vi "mod_sub_phase noise fit.vi"(0 "raw phase noise in":dbl[](array[numeric]) format="%.2f", 3 "f0":dbl=100.0 format="%.2f", 4 "error in (no error)":errorcluster, 5 "df":dbl=99.99921875610347 format="%.2f", 6 "polynomial order":i32=5, 7 "Section at what multiples?":dbl=10.0 format="%.2f", 9 "multiple buffer?":dbl=2.0 format="%.2f") -> (14 "phase noise fit":dbl[](array[numeric]) format="%.2f", 17 "phase noise plots":T1(array[cluster]) {"phase noise" format="%.2f"; "Ramp Pattern" format="%.2f"}, 19 "error out":errorcluster)   [LabVIEW 2020, in "niAMT.lvlib"]
uses:
  <vilib>/addons/Modulation/niAMT.lvlib
  <vilib>/Analysis/1siggen.llb/Ramp Pattern by Samples.vi
  <vilib>/measure/NI_MABase.lvlib
  <vilib>/Analysis/NI_AALBase.lvlib
  <vilib>/Analysis/NI_AALPro.lvlib
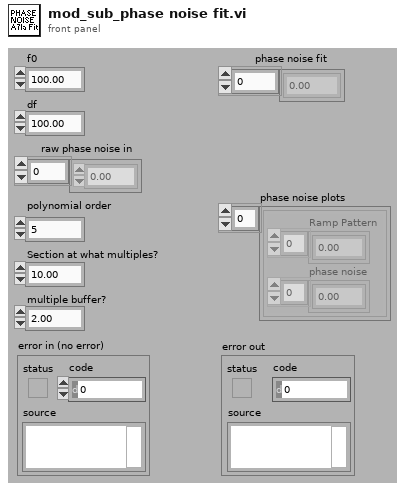
[diagram p1: front panel]
types:
  T1 = cluster{"Ramp Pattern":dbl[], "phase noise":dbl[]}[]
  T2 = enum32{"SVD", "Givens", "Givens2", "Householder", "LU Decomposition", "Cholesky"}
  T3 = cluster{"Ramp Pattern":dbl[], "raw phase noise in":dbl[]}
  T4 = cluster{"Ramp Pattern":dbl[], "raw phase noise in":dbl[]}[]
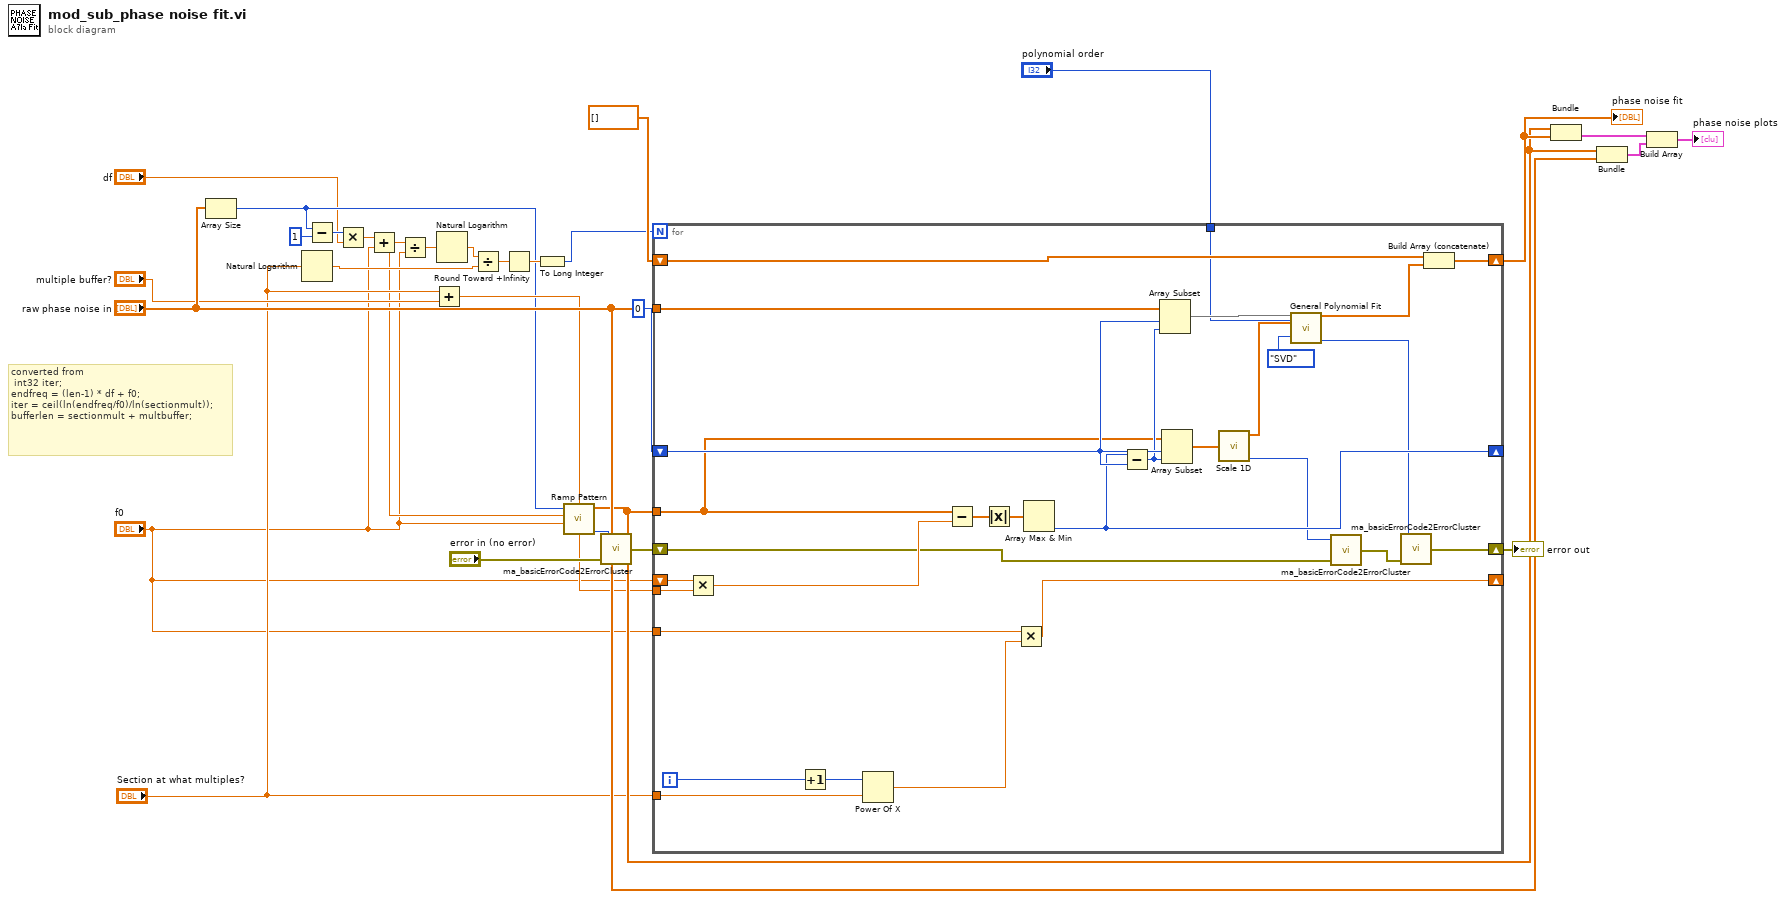
[diagram p0: block diagram]
diagram:
  # "converted from\n int32 iter;\nendfreq = (len-1) * df + f0;\niter = ceil(ln(endfreq/f0)/ln(sectionmult));\nbufferlen = sectionmult + multbuffer;"
  n1 = Array Size(array="raw phase noise in") -> (size(s)=w2:i32)
  n2 = Natural Logarithm(1:"Section at what multiples?") -> (0:w11:dbl)
  n3 = Subtract(x=w2, y=1) -> (x-y=w15:i32)
  n4 = Multiply(x=w15, y="df") -> (x*y=w14:dbl)
  n5 = Add(x=w14, y="f0") -> (x+y=w4:dbl)
  n6 = Divide(x=w4, y="f0") -> (x/y=w13:dbl)
  n7 = Add(x="Section at what multiples?", y="multiple buffer?") -> (x+y=w7:dbl)
  n8 = Natural Logarithm(1:w13) -> (0:w12:dbl)
  n9 = Divide(x=w12, y=w11) -> (x/y=w10:dbl)
  n10 = Round Toward +Infinity(x=w10) -> (ceil(x): smallest int >= x=w9:dbl)
  n11 = To Long Integer(number=w9) -> (32bit integer=w8:i32)
  n12 = call-poly <vilib>:"Ramp Pattern.vi"("start"="f0", "end"=w4, "samples"=w2) -> ("error"=w20:i32, "Ramp Pattern"=w21:dbl[])  [unwired: 7 in]
  n13 = call <vilib>:"ma_basicErrorCode2ErrorCluster.vi"("error in (no error)"="error in (no error)", "Error Code"=w20) -> ("error out"=w19:errorcluster)  [unwired: 1 in]
  n14 = for {
    N: w8 -> [_]
    shift-right: [w38] -> _
    shift-left: 0 -> [w54]
    tunnel: "raw phase noise in" -> [w55]
    tunnel: w21 -> [w45]
    tunnel: "Section at what multiples?" -> [w42]
    tunnel: "f0" -> [w58]
    tunnel: w7 -> [w56]
    shift-right: [w57] -> _
    shift-left: "f0" -> [w40]
    shift-right: [w49] -> w25
    shift-left: dbl[] [] -> [w48]
    tunnel: "polynomial order" -> [w36]
    shift-right: [w30] -> w18
    shift-left: w19 -> [w31]
    i -> [w44]
    n15 = Multiply(x=w40, y=w56) -> (x*y=w39:dbl)
    n16 = Increment(x=w44) -> (x+1=w43:i32)
    n17 = Power Of X(1:w42, 2:w43) -> (0:w41:dbl)
    n18 = Subtract(x=w45, y=w39) -> (x-y=w47:dbl[])
    n19 = Absolute Value(x=w47) -> (abs(x)=w46:dbl[])
    n20 = Multiply(x=w58, y=w41) -> (x*y=w57:dbl)
    n21 = Array Max & Min(array=w46) -> (min index (indices)=w38:i32)  [unwired: 3 out]
    n22 = Subtract(x=w38, y=w54) -> (x-y=w53:i32)
    n23 = Array Subset(array=w55, index=w54, length=w53) -> (w52:dbl[])
    n24 = Array Subset(array=w45, index=w54, length=w53) -> (w51:dbl[])
    n25 = call <vilib>:"Scale 1D.vi"("X"=w51) -> ("Y=(X-offset)/scale"=w35:dbl[], "error"=w32:i32)  [unwired: 2 out]
    n26 = call <vilib>:"General Polynomial Fit.vi"("Y"=w52, "polynomial order"=w36, "X"=w35, "algorithm"=T2."SVD") -> ("Best Polynomial Fit"=w37:dbl[], "error"=w34:i32)  [unwired: 8 in, 2 out]
    n27 = call <vilib>:"ma_basicErrorCode2ErrorCluster.vi"("error in (no error)"=w31, "Error Code"=w32) -> ("error out"=w33:errorcluster)  [unwired: 1 in]
    n28 = call <vilib>:"ma_basicErrorCode2ErrorCluster.vi"("error in (no error)"=w33, "Error Code"=w34) -> ("error out"=w30:errorcluster)  [unwired: 1 in]
    n29 = Build Array (concatenate)(w48, w37) -> (w49:dbl[])
  }
  "phase noise fit" <- w25
  "error out" <- w18
  n30 = Bundle("Ramp Pattern"=w21, w25) -> (w22:cluster{"Ramp Pattern":dbl[], dbl[]})  [unwired: 1 out]
  n31 = Bundle("Ramp Pattern"=w21, "raw phase noise in"="raw phase noise in") -> (w26:T3)  [unwired: 1 out]
  n32 = Build Array(w22, w26) -> (→"phase noise plots":T4)
